vi "Temperature_Conversion.vi"() -> ()   [LabVIEW 2019]
panel:
  in  "To: Unit":enum16{"F", "C", "K"}(ring)
  in  "From: Unit":enum16{"F", "C", "K"}(ring)
  in  "Convert Button":bool
  in  "Exit Button":bool
  out "Your Result":dbl
  in  "Input a value":i32
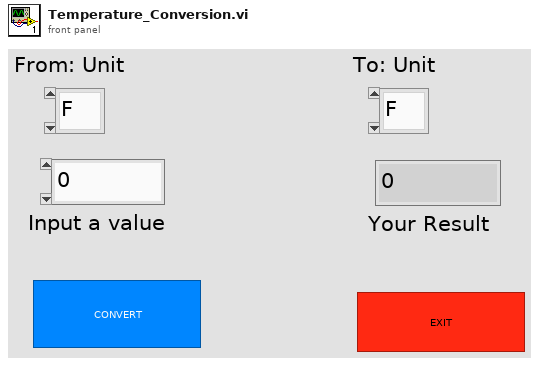
[diagram p1: front panel]
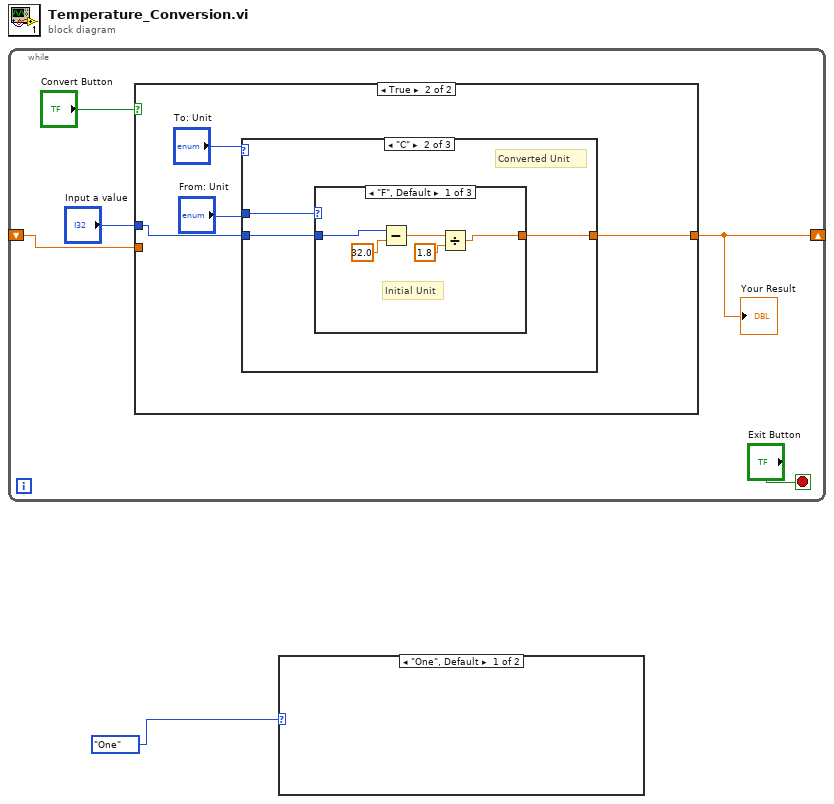
[diagram p0: block diagram]
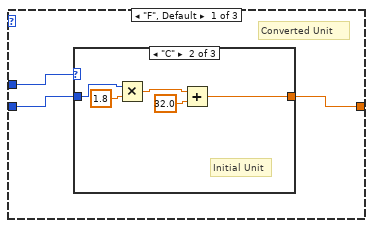
[diagram p4: hidden frame]
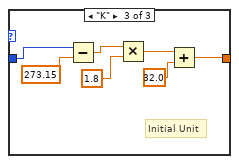
[diagram p6: hidden frame]
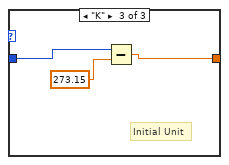
[diagram p8: hidden frame]
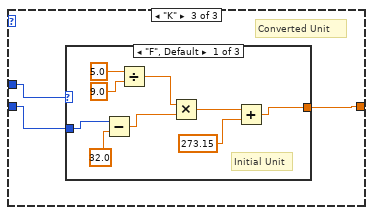
[diagram p9: hidden frame]
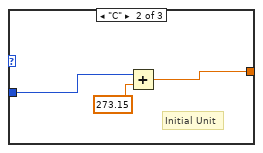
[diagram p10: hidden frame]
diagram:
  n1 = while {
    shift-right: [w2] -> _
    shift-left: _ -> [w3]
    stop <- "Exit Button" stop-if-true
    n2 = case shown="True" "Convert Button" {
      tunnel: "Input a value" -> [_ w11]
      tunnel: [w7 w10] -> w2
      tunnel: w3 -> [w7 _]
      frame False {
      }
      frame True {
        n3 = case shown="\"C\"" "To: Unit" {
          tunnel: "From: Unit" -> [w14 w30 w42]
          tunnel: w11 -> [w13 w29 w41]
          tunnel: [w12 w28 w40] -> w10
          frame "F", Default {
            # "Converted Unit"
            n4 = case shown="\"C\"" w14 {
              tunnel: w13 -> [w15 w17 w26]
              tunnel: [w15 w16 w23] -> w12
              frame "F", Default {
                # "Same Unit so no change"
                # "Initial Unit"
              }
              frame "C" {
                # "Initial Unit"
                n5 = Multiply(x=w17, y=1.8) -> (x*y=w18:dbl)
                n6 = Add(x=w18, y=32.0) -> (x+y=w16:dbl)
              }
              frame "K" {
                # "Initial Unit"
                n7 = Subtract(x=w26, y=273.15) -> (x-y=w24:dbl)
                n8 = Multiply(x=w24, y=1.8) -> (x*y=w21:dbl)
                n9 = Add(x=w21, y=32.0) -> (x+y=w23:dbl)
              }
            }
          }
          frame "C" {
            # "Converted Unit"
            n10 = case shown="\"F\", Default" w30 {
              tunnel: w29 -> [w31 w36 w38]
              tunnel: [w35 w36 w37] -> w28
              frame "F", Default {
                # "Initial Unit"
                n11 = Subtract(x=w31, y=32.0) -> (x-y=w33:dbl)
                n12 = Divide(x=w33, y=1.8) -> (x/y=w35:dbl)
              }
              frame "C" {
                # "Same Unit so no change"
                # "Initial Unit"
              }
              frame "K" {
                # "Initial Unit"
                n13 = Subtract(x=w38, y=273.15) -> (x-y=w37:dbl)
              }
            }
          }
          frame "K" {
            # "Converted Unit"
            n14 = case shown="\"F\", Default" w42 {
              tunnel: w41 -> [w50 w53 w55]
              tunnel: [w43 w52 w55] -> w40
              frame "F", Default {
                # "Initial Unit"
                n15 = Subtract(x=w50, y=32.0) -> (x-y=w46:dbl)
                n16 = Divide(x=5.0, y=9.0) -> (x/y=w47:dbl)
                n17 = Multiply(x=w47, y=w46) -> (x*y=w45:dbl)
                n18 = Add(x=w45, y=273.15) -> (x+y=w43:dbl)
              }
              frame "C" {
                # "Initial Unit"
                n19 = Add(x=w53, y=273.15) -> (x+y=w52:dbl)
              }
              frame "K" {
                # "Same Unit so no change"
                # "Initial Unit"
              }
            }
          }
        }
      }
    }
    "Your Result" <- w2
  }
  n20 = case shown="\"One\", Default" enum16{"One", "Two", "Tree"}."One" {
    frame "One", Default {
    }
    frame "Two" {
    }
  }
